vi "CH_LM Config Trend Zoom.vi"(0 "Meter Index":i32, 3 "Zoom Mode (1)":T1=enum."1", 5 "error in (no error)":errorcluster, 7 "Timeout / ms (3000)":i32=1000, 8 "Action (query)":bool, 9 "Lock Timeout / ms (1000)":i32=1000) -> (11 "Lock timed out":bool, 14 "Meter Index":i32, 17 "Zoom Mode":T1=enum."1", 19 "error out":errorcluster)   [LabVIEW 2012, in "CH_LM.lvlib"]
doc: "This VI will query or set measurement mode and unit.\n\n<B>Attention:</B> The command will be ignored when an optical probe is attached or if a valid probe is not attached."
uses:
  CH_LM.lvlib
  CH_LM Zoom Factor.ctl
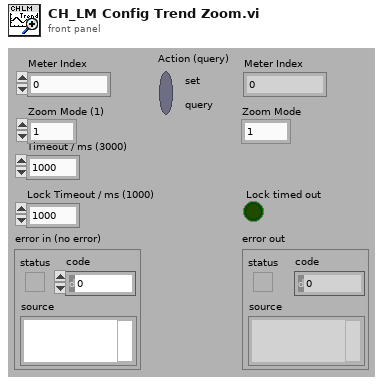
[diagram p1: front panel]
types:
  T1 = typedef "CH_LM.lvlib/CH_LM Zoom Factor.ctl" = enum16{"Auto", "1", "2", "5", "10", "20"}
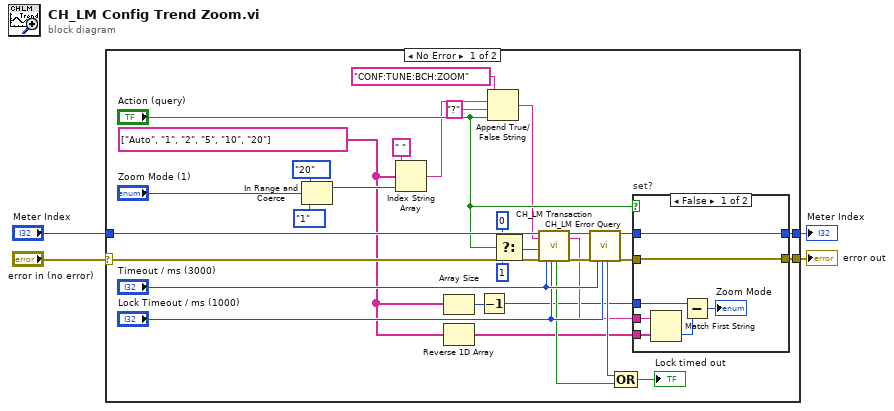
[diagram p0: block diagram]
diagram:
  n1 = case shown="No Error" "error in (no error)" {
    selector: "error in (no error)" -> [w35 w46]
    tunnel: [w33 w46] -> w4
    tunnel: "Meter Index" -> [w34 w45]
    tunnel: [w32 w45] -> w1
    frame No Error {
      w7 = string[] ["Auto", "1", "2", "5", "10", "20"]
      n2 = In Range and Coerce(upper limit=enum16{"Auto", "1", "2", "5", "10", "20"}."20", x="Zoom Mode (1)", lower limit=enum16{"Auto", "1", "2", "5", "10", "20"}."1" ("f")) -> (coerced(x)=w17:T1)  [unwired: 1 out]
      n3 = Index String Array(1:w17, 2:w7, 3:" " ("string (\"\")")) -> (0:w16:string)
      n4 = Array Size(array=w7) -> (size(s)=w6:i32)
      n5 = Reverse 1D Array(array=w7) -> (reversed array=w8:string[])
      n6 = Decrement(x=w6) -> (x-1=w5:i32)
      n7 = Append True/False String(1:"Action (query)", 2:"?" ("true string"), 3:w16, 4:"CONF:TUNE:BCH:ZOOM" ("Command String")) -> (0:w15:string)
      n8 = Select(t=0, s="Action (query)", f=1 ("NofStrings (-1:all)")) -> (s? t:f=w19:i32)
      n9 = call "CH_LM Transaction.vi"("Meter Index"=w34, "Command String"=w15, "NofStrings (-1:all)"=w19, "error in (no error)"=w35, "Timeout / ms (3000)"="Timeout / ms (3000)", "Lock Timeout / ms (1000)"="Lock Timeout / ms (1000)") -> ("Lock timed out"=w23:bool, "Meter Index"=w14:i32, "Response"=w12:string, "error out"=w13:errorcluster)  [unwired: 10 out]
      n10 = call "CH_LM Error Query.vi"("Meter Index"=w14, "error in (no error)"=w13, "Timeout / ms (3000)"="Timeout / ms (3000)", "Lock Timeout / ms (1000)"="Lock Timeout / ms (1000)") -> ("Lock timed out"=w24:bool, "Meter Index"=w26:i32, "error out"=w25:errorcluster)  [unwired: 13 out]
      n11 = Compound Arithmetic op=OR(w24, w23) -> (→"Lock timed out":bool)
      n12 = case "set?" shown="False" "Action (query)" {
        tunnel: w25 -> [w41 w44]
        tunnel: [w41 w44] -> w33
        tunnel: w26 -> [w42 w43]
        tunnel: [w42 w43] -> w32
        tunnel: w12 -> [w40 _]
        tunnel: w8 -> [w39 _]
        tunnel: w5 -> [w38 _]
        frame False {
          n13 = Match First String(2:w39, 3:w40) -> (0:w37:i32)  [unwired: 1 out]
          n14 = Subtract(x=w38, y=w37) -> (x-y=→"Zoom Mode":i32)
        }
        frame True {
        }
      }
    }
    frame Error {
    }
  }
  "error out" <- w4
  "Meter Index" <- w1
